vi "tmp-move-and-glueDispenser.vi"() -> ()   [LabVIEW 2016]
uses:
  Classes/Controllers/Motion/Copy of Motion Folder/Motion.lvclass
  Classes/Controllers/Camera/Copy of Controller Folder/Controller.lvclass
  Classes/Controllers/I-O/Copy of NI-DAQ Folder/NI-DAQ.lvclass
  <vilib>/Utility/file.llb/Read Delimited Spreadsheet (DBL).vi
  Control 1.ctl
panel:
  out "HDI rotaion r-phi":dbl[](array[numeric])
  in  "values 2":bool[](array[boolean])=[FALSE]
  in  "values":bool[](array[boolean])=[TRUE]
  in  "indices":i32[](array[numeric])=[0]
  in  "DAQ Module":i32
  out "millisecond timer value 2":u32
  out "millisecond timer value 3":u32
  out "millisecond timer value":u32
  out "Gantry Position":dbl[](array[numeric])
  out "pad center":T1[](array[typedef])
  out "default chip and sensor position w.r.t. 1st mark":dbl[][](array[numeric])
  in  "Defaul Residual Mark 1":T2[](array[typedef])=[1105.14, 602.336, 91.0863, 0.1]
  in  "Defaul Residual Mark 2":dbl[](array[numeric])=[1128.53, 833.788, 91.1726, 0.1]
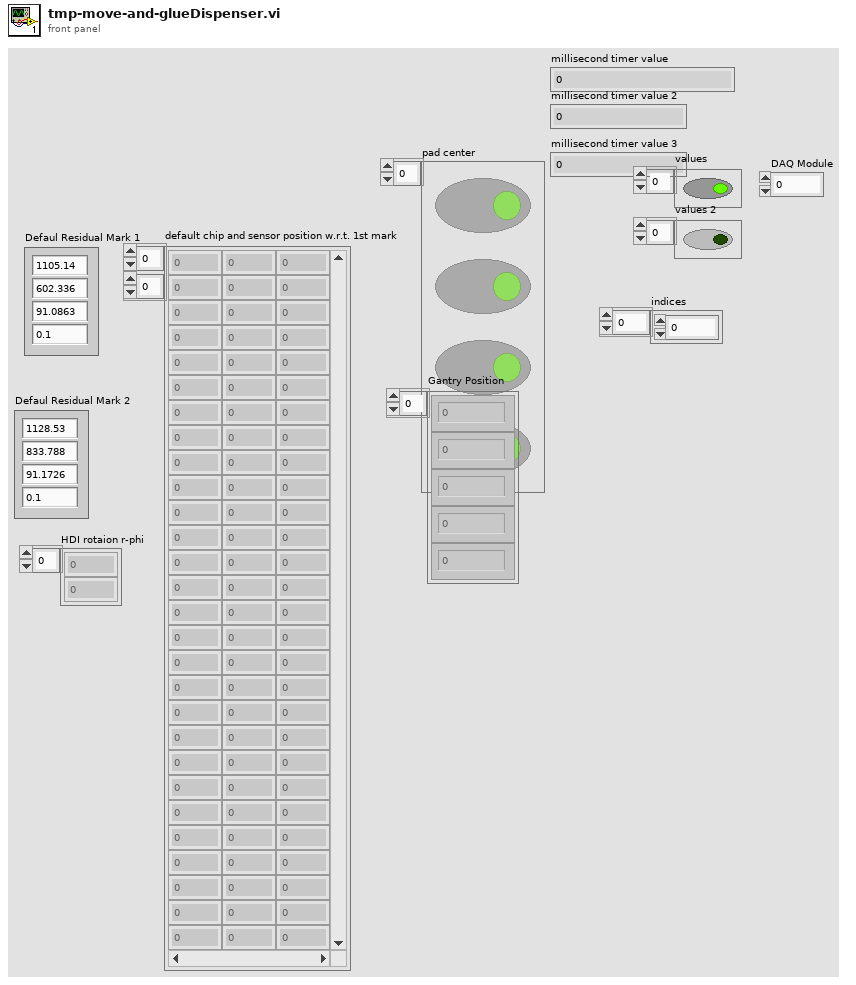
[diagram p1: front panel]
types:
  T1 = typedef "Control 1.ctl" = bool
  T2 = typedef "Control 1.ctl" = dbl
  T3 = typedef "Controller.lvclass/Controllers.ctl" = cluster{"Copy of Motion.lvclass":refnum<class "Motion.lvclass">, "Copy of I-O.lvclass":refnum<class "I-O.lvclass">, "Copy of Dispenser.lvclass":refnum<class "Dispenser.lvclass">}
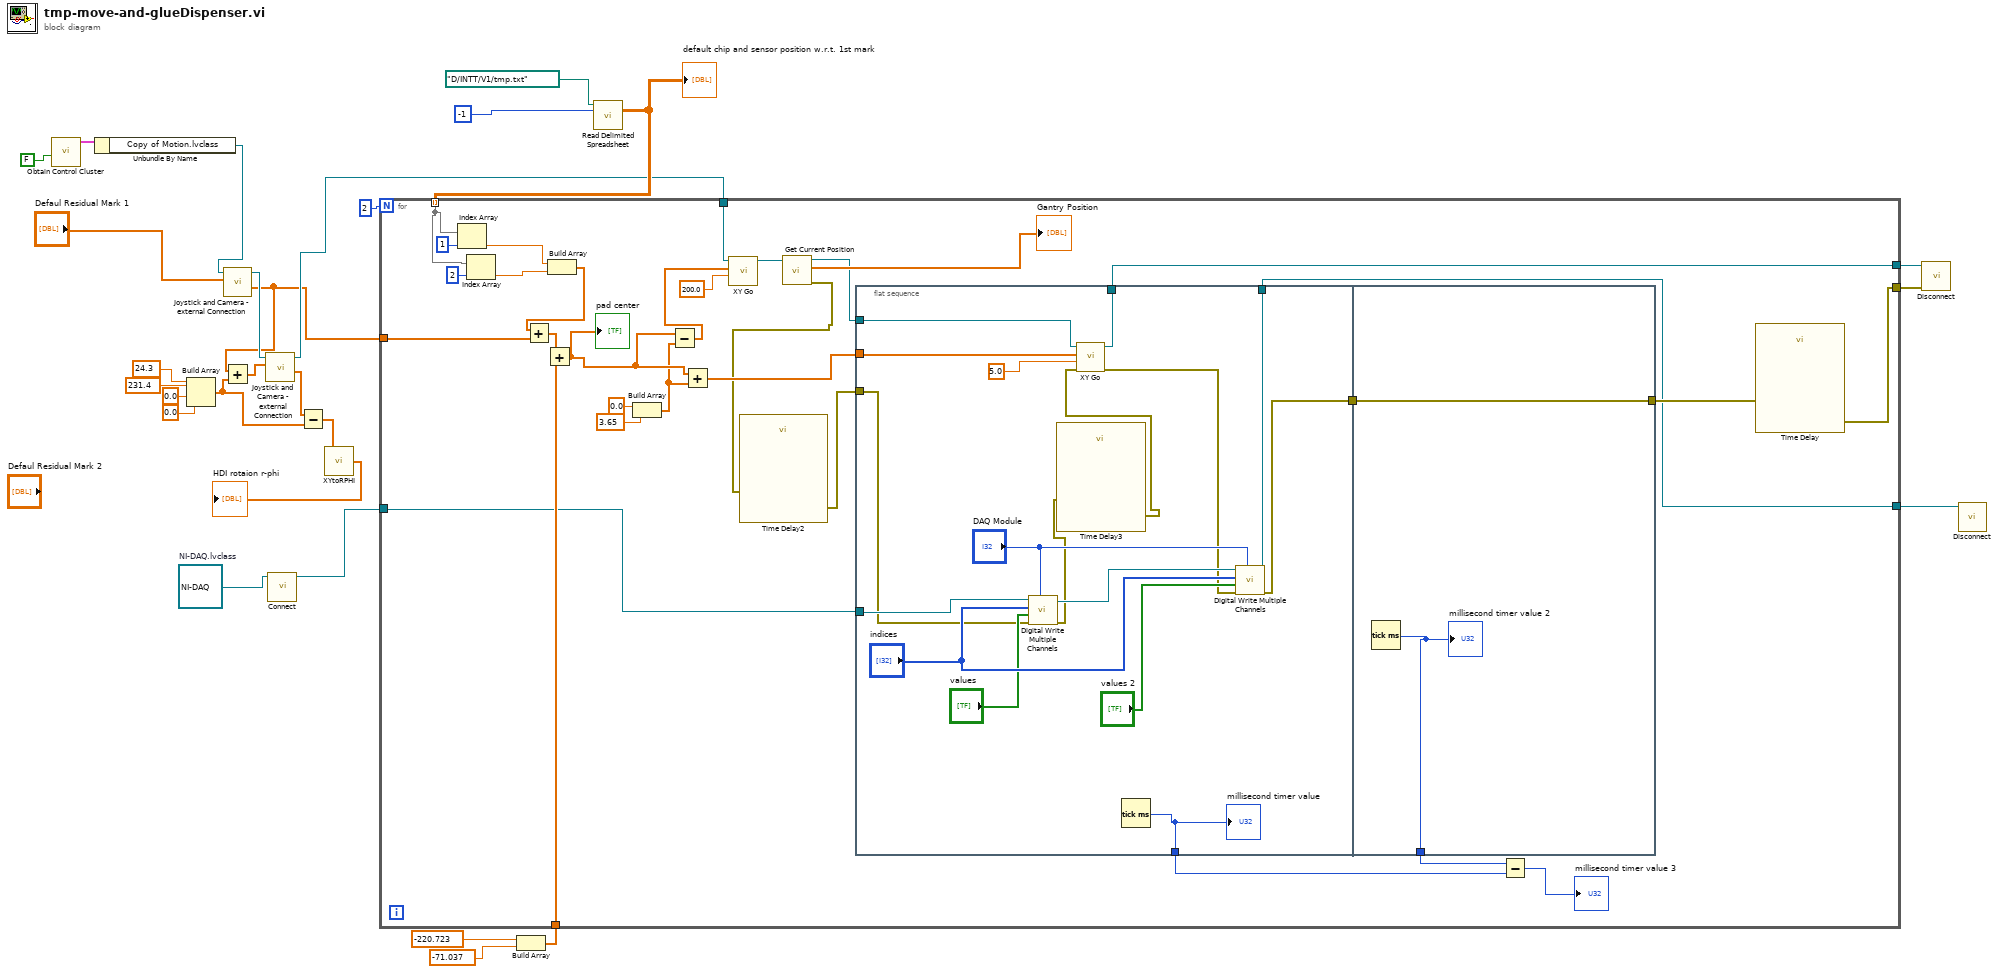
[diagram p0: block diagram]
diagram:
  w17 = refnum<class "NI-DAQ.lvclass"> refnum  # NI-DAQ.lvclass
  n1 = call "Obtain Control Cluster.vi"("I/O"=FALSE) -> ("Control Out"=w23:T3)  [unwired: 10 in]
  n2 = Unbundle By Name(w23) -> ("Copy of Motion.lvclass"=w14:refnum<class "Motion.lvclass">)
  n3 = Build Array(24.3 ("element"), 231.4 ("element"), 0.0 ("element"), 0.0 ("element")) -> (w3:dbl[])
  n4 = call "Joystick and Camera - external Connection.vi"("Motion in"=w14, "XYZTheta"="Defaul Residual Mark 1") -> ("Motion out"=w12:refnum<class "Motion.lvclass">, "Gantry"=w6:dbl[])  [unwired: 5 in, 2 out]
  n5 = Add(x=w6, y=w3) -> (x+y=w5:dbl[])
  n6 = call "Joystick and Camera - external Connection.vi"("Motion in"=w12, "XYZTheta"=w5) -> ("Motion out"=w11:refnum<class "Motion.lvclass">, "Gantry"=w4:dbl[])  [unwired: 5 in, 2 out]
  n7 = call-dynamic "Connect.vi"("NI-DAQ in"=w17) -> ("NI-DAQ out"=w16:refnum<class "NI-DAQ.lvclass">)  [unwired: 9 in, 1 out]
  n8 = Subtract(x=w4, y=w3) -> (x-y=w2:dbl[])
  n9 = call "XYtoRPHI.vi"("X-Y"=w2) -> ("r-phi"=→"HDI rotaion r-phi":dbl[])
  n10 = Build Array(-220.723, -71.037) -> (w18:dbl[])
  n11 = call-poly <vilib>:"Read Delimited Spreadsheet.vi"("file path (dialog if empty)"=path "D:/INTT/V1/tmp.txt", "number of rows (all:-1)"=-1) -> ("all rows"=w25:dbl[][])  [unwired: 8 in, 5 out]
  "default chip and sensor position w.r.t. 1st mark" <- w25
  n12 = for {
    N: 2 -> [_]
    tunnel: w25 -> [w57] mode=indexing
    tunnel: w6 -> [w53]
    tunnel: w11 -> [w52]
    tunnel: [w37] -> w22
    tunnel: [w41] -> w21
    tunnel: w18 -> [w50]
    tunnel: w16 -> [w30]
    tunnel: [w29] -> w15
    n13 = Index Array(array=w57, index=1) -> (element=w56:dbl)
    n14 = Index Array(array=w57, index=2) -> (element=w55:dbl)
    n15 = Build Array(w56, w55) -> (w54:dbl[])
    n16 = Add(x=w54, y=w53) -> (x+y=w49:dbl[])
    n17 = Add(x=w49, y=w50) -> (x+y=w44:dbl[])
    "pad center" <- w44
    n18 = Build Array(0.0 ("element"), 3.65 ("element")) -> (w43:dbl[])
    n19 = Subtract(x=w44, y=w43) -> (x-y=w42:dbl[])
    n20 = Add(x=w44, y=w43) -> (x+y=w39:dbl[])
    n21 = call-dynamic "XY Go.vi"("Speed"=200.0, "XY"=w42, "Motion in"=w52) -> ("Motion out"=w48:refnum<class "Motion.lvclass">)  [unwired: 7 in, 1 out]
    n22 = call-dynamic "Get Current Position.vi"("Motion in"=w48) -> ("error out"=w36:errorcluster, "XYZTheta Out"=→"Gantry Position":dbl[], "Motion out"=w40:refnum<class "Motion.lvclass">)  [unwired: 8 in]
    n23 = call "Time Delay2"("error in (no error)"=w36) -> ("error out"=w35:errorcluster)  [unwired: 10 in]
    n24 = flat-sequence {
      tunnel: [w73] -> w37
      tunnel: [w61] -> w33
      tunnel: w40 -> [w76]
      tunnel: w39 -> [w75]
      tunnel: w35 -> [w65]
      tunnel: [w72] -> w31
      tunnel: w30 -> [w66]
      tunnel: [w60] -> w29
      tunnel: [w78] -> w38
      tunnel: w33 -> [w78]
      tunnel: [w77] -> w32
      frame #0 {
        n25 = call-dynamic "Digital Write Multiple Channels.vi"("DAQ Module"="DAQ Module", "error in (no error)"=w65, "Values"="values", "Indices"="indices", "NI-DAQ in"=w66) -> ("error out"=w64:errorcluster, "NI-DAQ out"=w70:refnum<class "NI-DAQ.lvclass">)  [unwired: 5 in]
        n26 = call "Time Delay3"("error in (no error)"=w64) -> ("error out"=w63:errorcluster)  [unwired: 10 in]
        n27 = call-dynamic "XY Go.vi"("error in (no error)"=w63, "Speed"=5.0, "XY"=w75, "Motion in"=w76) -> ("error out"=w62:errorcluster, "Motion out"=w73:refnum<class "Motion.lvclass">)  [unwired: 6 in]
        n28 = Tick Count (ms)() -> (millisecond timer value=w72:u32)
        "millisecond timer value" <- w72
        n29 = call-dynamic "Digital Write Multiple Channels.vi"("DAQ Module"="DAQ Module", "error in (no error)"=w62, "Values"="values 2", "Indices"="indices", "NI-DAQ in"=w70) -> ("error out"=w61:errorcluster, "NI-DAQ out"=w60:refnum<class "NI-DAQ.lvclass">)  [unwired: 5 in]
      }
      frame #1 {
        n30 = Tick Count (ms)() -> (millisecond timer value=w77:u32)
        "millisecond timer value 2" <- w77
      }
    }
    n31 = Subtract(x=w32, y=w31) -> (x-y=→"millisecond timer value 3":u32)
    n32 = call "Time Delay"("error in (no error)"=w38) -> ("error out"=w41:errorcluster)  [unwired: 10 in]
  }
  n33 = call-dynamic "Disconnect.vi"("error in (no error)"=w21, "Controller in"=w22) -> ()  [unwired: 8 in, 1 out]
  n34 = call-dynamic "Disconnect.vi"("I-O in"=w15) -> ()  [unwired: 9 in, 1 out]
